vi "traffic-ligths.vi"() -> ()   [LabVIEW 2025]
panel:
  out "green":bool
  out "yel":bool
  out "red":bool
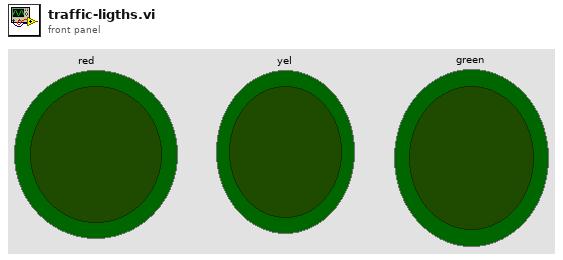
[diagram p1: front panel]
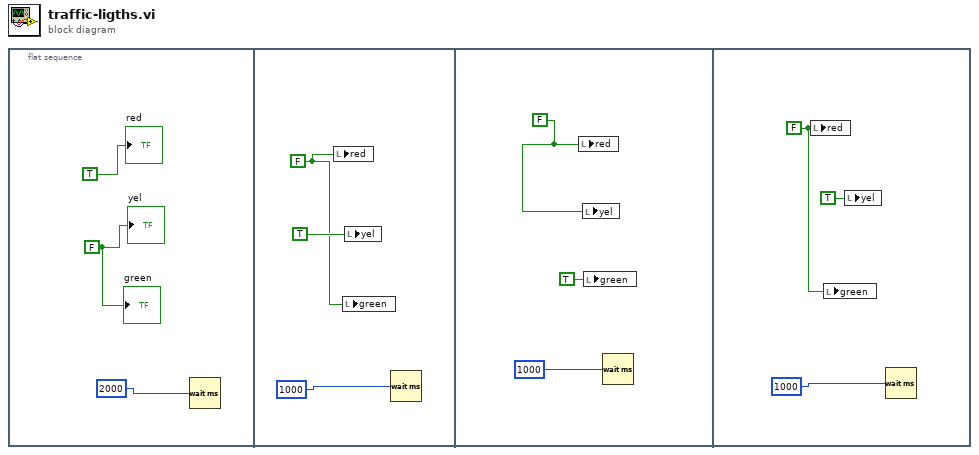
[diagram p0: block diagram]
diagram:
  n1 = flat-sequence {
    frame #0 {
      w2 = FALSE ("yel")
      n2 = Wait (ms)(milliseconds to wait=2000) -> ()  [unwired: 1 out]
      "red" <- TRUE ("red")
      "yel" <- w2
      "green" <- w2
    }
    frame #1 {
      w4 = FALSE ("red")
      n3 = local write "red"(w4) -> ()
      n4 = local write "green"(w4) -> ()
      n5 = local write "yel"(TRUE ("yel")) -> ()
      n6 = Wait (ms)(milliseconds to wait=1000) -> ()  [unwired: 1 out]
    }
    frame #2 {
      w9 = FALSE
      n7 = local write "red"(w9) -> ()
      n8 = local write "yel"(w9) -> ()
      n9 = local write "green"(TRUE ("green")) -> ()
      n10 = Wait (ms)(milliseconds to wait=1000) -> ()  [unwired: 1 out]
    }
    frame #3 {
      w11 = FALSE ("red")
      n11 = local write "red"(w11) -> ()
      n12 = local write "green"(w11) -> ()
      n13 = local write "yel"(TRUE ("yel")) -> ()
      n14 = Wait (ms)(milliseconds to wait=1000) -> ()  [unwired: 1 out]
    }
  }
